vi "PhaseShifter demo Main.vi"   [LabVIEW 2020]
panel:
  # "Digital Phase Shifter, 3.5GHz"
types:
  T1 = enum32{"Invalid", "Standard", "Closed", "Hidden", "Minimized", "Maximized"}
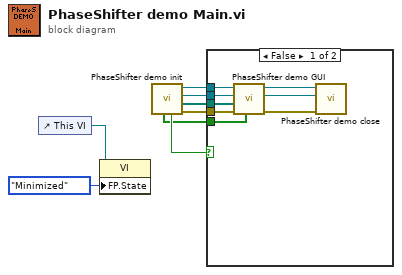
[diagram p0: block diagram]
diagram:
  n1 = control-ref of="This VI"() -> (w2:refnum<vi>)
  n2 = property class="VI"(reference=w2, "FP.State"=T1."Minimized" ("Front Panel Window:State")) -> ()  [unwired: 1 in, 2 out]
  n3 = call "PhaseShifter demo init.vi"() -> ("Error Out"=w8:errorcluster, "De-embedding files"=w5:path[], "Toggle 6.lvclass"=w6:refnum<class "Toggle 6.lvclass">, "Vector Network Analyzer.lvclass"=w7:refnum<class "Vector Network Analyzer.lvclass">, "Cancelled"=w4:bool, "VNA ports 2"=w3:bool[])  [unwired: 6 in]
  n4 = case shown="False" w4 {
    tunnel: w8 -> [w16 _]
    tunnel: w7 -> [w15 _]
    tunnel: w6 -> [w12 _]
    tunnel: w5 -> [w10 _]
    tunnel: w3 -> [w9 _]
    frame False {
      n5 = call "PhaseShifter demo GUI.vi"("VNA ports"=w9, "Error In"=w16, "De-embedding files"=w10, "Toggle 6.lvclass"=w12, "Vector Network Analyzer.lvclass"=w15) -> ("Error Out"=w14:errorcluster, "Toggle 6.lvclass 2"=w11:refnum<class "Toggle 6.lvclass">, "Vector Network Analyzer.lvclass 2"=w13:refnum<class "Vector Network Analyzer.lvclass">)  [unwired: 4 in]
      n6 = call "PhaseShifter demo close.vi"("Error In"=w14, "Toggle 6.lvclass"=w11, "Vector Network Analyzer.lvclass"=w13) -> ()  [unwired: 8 in, 1 out]
    }
    frame True {
    }
  }
